vi "_user.vi"(8 "error in (no error)":errorcluster, 10 "Send":string="Command", 11 "VISA resource name":refnum<visa-resource-name>="COM1") -> (0 "error out":errorcluster, 2 "Answer":string="Command", 3 "VISA resource name":refnum<visa-resource-name>="COM1")   [LabVIEW 2017]
panel:
  # "Dummy user VI to communicate with instruments (voltmeter, gaussmeter, temperature sensor...)"
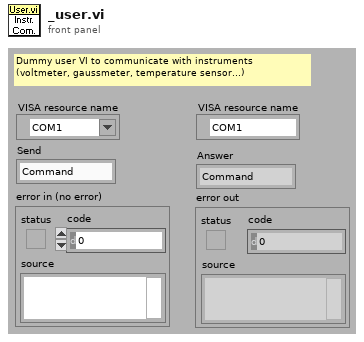
[diagram p1: front panel]
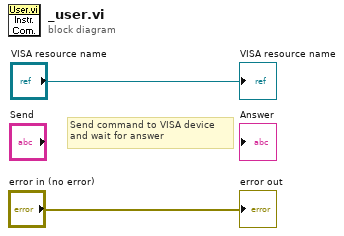
[diagram p0: block diagram]
diagram:
  # "Send command to VISA device\nand wait for answer"
  "error out" <- "error in (no error)"
  "VISA resource name" <- "VISA resource name"
